vi "Get Completion.vi"(0 "ICM Ref In":refnum<class "Modbus Master.lvclass">, 11 "error in (no error)":errorcluster) -> (4 "ICM Ref Out":refnum<class "Modbus Master.lvclass">, 6 "Completion %":dbl, 15 "error out":errorcluster)   [LabVIEW 2024]
uses:
  <vilib>/NI/Modbus Library/API/Master/Modbus Master.lvclass
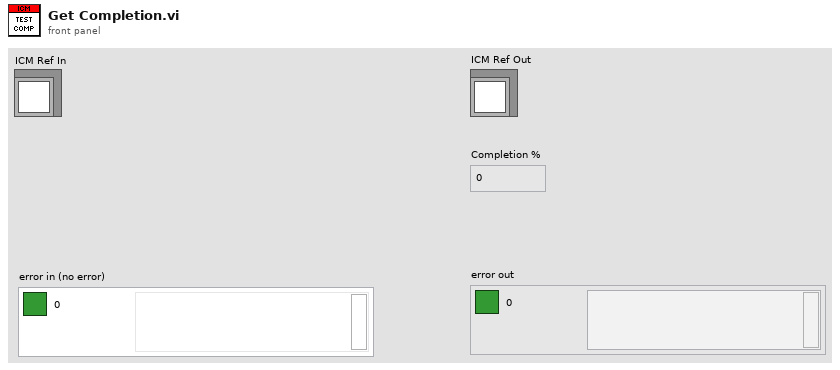
[diagram p1: front panel]
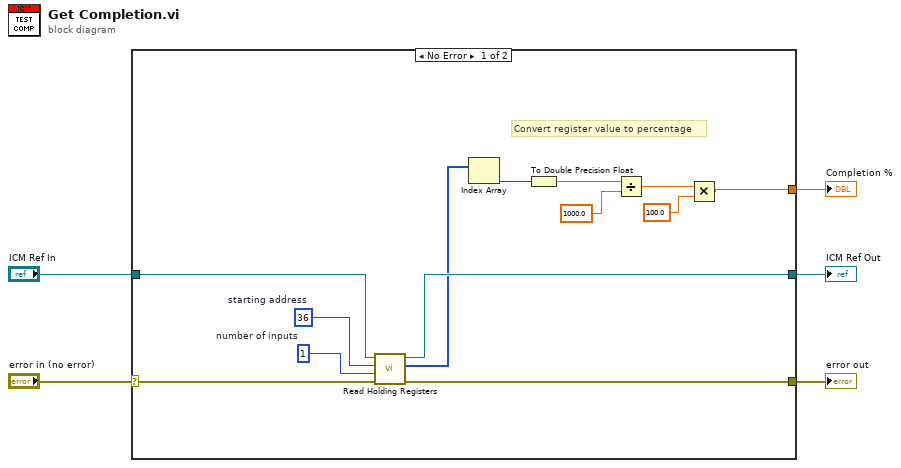
[diagram p0: block diagram]
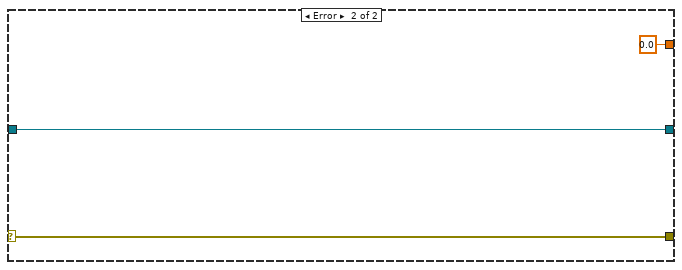
[diagram p2: hidden frame]
diagram:
  n1 = case shown="No Error" "error in (no error)" {
    selector: "error in (no error)" -> [w18 w20]
    tunnel: [w17 w20] -> w5
    tunnel: "ICM Ref In" -> [w16 w21]
    tunnel: [w13 w21] -> w2
    tunnel: [w7 0.0] -> w1
    frame No Error {
      w14 = u16 1  # number of inputs
      w15 = u16 36  # starting address
      # "Convert register value to percentage"
      n2 = call-dynamic "Read Holding Registers.vi"("error in"=w18, "number of inputs"=w14, "starting address"=w15, "Modbus master in"=w16) -> ("error out"=w17:errorcluster, "register values"=w12:u16[], "Modbus master out"=w13:refnum<class "Modbus Master.lvclass">)  [unwired: 5 in]
      n3 = Index Array(array=w12) -> (element=w11:u16)  [unwired: 1 in]
      n4 = To Double Precision Float(number=w11) -> (double precision float=w6:dbl)
      n5 = Divide(x=w6, y=1000.0) -> (x/y=w9:dbl)
      n6 = Multiply(x=w9, y=100.0) -> (x*y=w7:dbl)
    }
    frame Error {
    }
  }
  "error out" <- w5
  "ICM Ref Out" <- w2
  "Completion %" <- w1
